vi "Read Configuration.vi"(8 "error in (no error)":errorcluster, 11 "TroSpec in":refnum<class "PL ISTEQ TroSpec.lvclass">) -> (0 "error out":errorcluster, 2 "configuration":T1 {"gain" items=["1", "3", "5", "7"]; "period, s" format="%#_6p"}, 3 "TroSpec out":refnum<class "PL ISTEQ TroSpec.lvclass">)   [LabVIEW 2015, in "PL ISTEQ TroSpec.lvclass"]
doc: "Reads configuration."
uses:
  PL ISTEQ TroSpec.lvclass
  PL ISTEQ TroSpec.lvclass/PL ISTEQ TroSpec.ctl
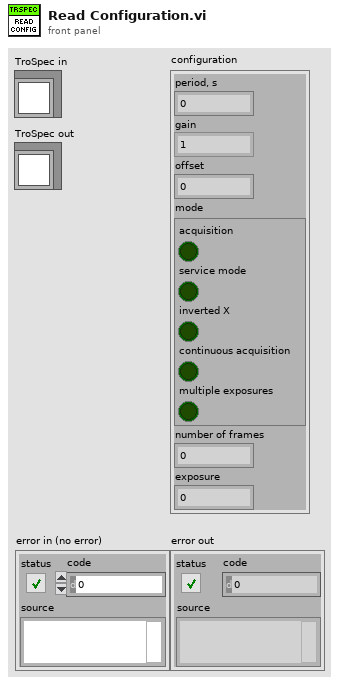
[diagram p1: front panel]
types:
  T1 = cluster{"period, s":dbl, "gain":u16, "offset":u16, "mode":cluster{"acquisition":bool, "service mode":bool, "inverted X":bool, "continuous acquisition":bool, "multiple exposures":bool}, "number of frames":u32, "exposure":u32}
  T2 = cluster{"Boolean array[0]":bool, "Boolean array[1]":bool, "Boolean array[2]":bool, "Boolean array[3]":bool, "Boolean array[4]":bool}
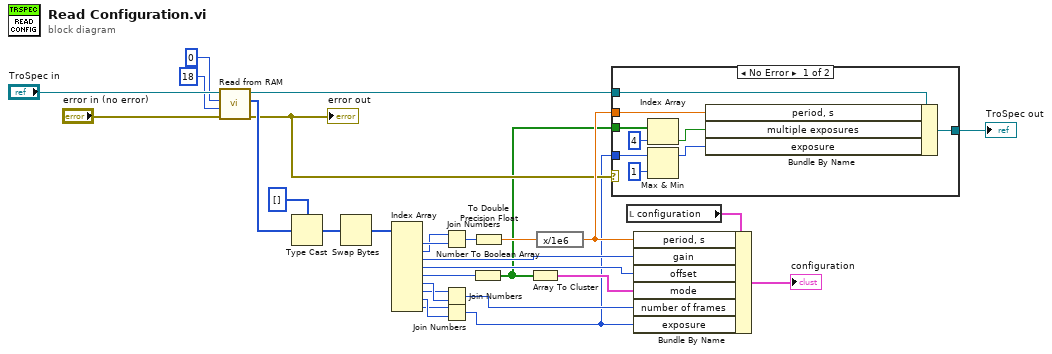
[diagram p0: block diagram]
diagram:
  n1 = call "Read from RAM.vi"("error in (no error)"="error in (no error)", "size"=u16 18, "address"=u16 0, "TroSpec in"="TroSpec in") -> ("error out"=w3:errorcluster, "data"=w22:u8[], "TroSpec out"=w6:refnum<class "PL ISTEQ TroSpec.lvclass">)  [unwired: 5 in]
  "error out" <- w3
  n2 = Type Cast(type=u16[] [] ("data"), x=w22) -> (*(type *) &x=w21:u16[])
  n3 = Swap Bytes(anything=w21) -> (byte swapped=w20:u16[])
  n4 = Index Array(array=w20) -> (element #1=w19:u16, element #2=w18:u16, element #3=w11:u16, element #4=w10:u16, element #5=w9:u16, element #6=w17:u16, element #7=w14:u16, element #8=w16:u16, element #9=w15:u16)  [unwired: 9 in]
  n5 = Join Numbers(hi=w18, lo=w19) -> ((hi.lo)=w13:u32)
  n6 = Join Numbers(hi=w14, lo=w17) -> ((hi.lo)=w7:u32)
  n7 = Join Numbers(hi=w15, lo=w16) -> ((hi.lo)=w1:u32)
  n8 = Number To Boolean Array(number=w9) -> (Boolean array=w2:bool[])
  n9 = To Double Precision Float(number=w13) -> (double precision float=w12:dbl)
  n10 = Array To Cluster(array=w2) -> (cluster=w8:T2)
  n11 = expression code="x/1e6"(w12) -> (w4:dbl)
  n12 = case shown="No Error" w3 {
    tunnel: w6 -> [w38 w39]
    tunnel: [w37 w39] -> w5
    tunnel: w4 -> [w36 _]
    tunnel: w2 -> [w35 _]
    tunnel: w1 -> [w32 _]
    frame No Error {
      n13 = Index Array(array=w35, index=4) -> (element=w33:bool)
      n14 = Max & Min(x=w32, y=u32 1) -> (max(x,y)=w31:u32)  [unwired: 1 out]
      n15 = Bundle By Name(cluster=w38, "period, s"=w36, "multiple exposures"=w33, "exposure"=w31) -> (w37:refnum<class "PL ISTEQ TroSpec.lvclass">)
    }
    frame Error {
    }
  }
  "TroSpec out" <- w5
  n16 = local read "configuration"() -> (w25:T1)
  n17 = Bundle By Name(cluster=w25, "period, s"=w4, "gain"=w11, "offset"=w10, "mode"=w8, "number of frames"=w7, "exposure"=w1) -> (→"configuration":T1)
